vi "AFG3352X.constructor.vi"(0 "name":string, 2 "data in":string, 5 "error in (no error)":errorcluster) -> (14 "i ref out":refnum<vi>, 16 "data out":string, 19 "error out":errorcluster)   [LabVIEW 2014, in "AFG3352X.lvlib"]
doc: "Constructor of the AG33XXX class.\n\nLicense Agreement for this software:\n\nCopyright (C)\nGesellschaft für Schwerionenforschung, GSI\nPlanckstr. 1\n64291 Darmstadt\nGermany\n\nContact: D.Beck@gsi.de \n\nThis program is free software; you can redistribute it and/or modify it under the terms of the \nGNU General Public License as published by the Free Software Foundation; either version 2 of \nthe license, or (at your option) any later version.\n\nThis program is distributed in the hope that it will be useful, but WITHOUT ANY WARRANTY; \nwithout even the implied warranty of MERCHANTABILITY or FITNESS FOR A PARTICULAR PURPOSE. See the GNU General License for more details (http://www.gnu.org).\n\nGesellschaft für Schwerionenforschung, GSI\nPlanckstr. 1, 64291 Darmstadt, Germany\nFor all questions and ideas contact: M.Richter@gsi.de, H.Brand@gsi.de or D.Beck@gsi.de.\nLast update: 16-JUN-2004"
uses:
  AFG3352X.lvlib
  CS_Core/CSApplicationBaseClasses/DeviceBase/DeviceBase.myEventNames.ctl
  CS_Core/CSApplicationBaseClasses/AFGBase/AFGBase.myEventNames.ctl
  CS_Core/CSSystem/CSSystemLib/CSSystemLib.lvlib
  CS_Core/CSApplicationBaseClasses/AFGBase/AFGBase.lvlib
  CS_Core/CSApplicationBaseClasses/DeviceBase/DeviceBase.lvlib
  CS_Core/CSObj/CSObj.lvlib
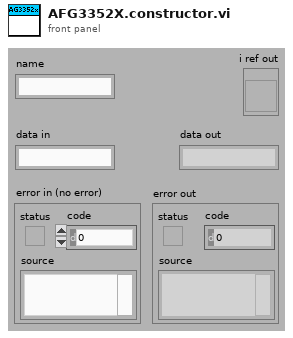
[diagram p1: front panel]
types:
  T1 = enum16{"SetAttribute", "GetAttribute", "CreateAttribute", "DestroyAttribute", "DestroyAllAtributes"}
  T2 = typedef "AFGBase.lvlib/AFGBase.myEventNames.ctl" = enum16{"lvmsg://SetFrequency", "lvmsg://GetFrequency", "lvmsg://SetAmplitude", "lvmsg://GetAmplitude", "lvmsg://SetPhase", "lvmsg://GetPhase", "lvmsg://SetDCOffset", "lvmsg://GetDCOffset", "lvmsg://SetWaveformType", "lvmsg://GetWaveformType", "lvmsg://SetOutputEnabled", "lvmsg://GetOutputEnabled", "lvmsg://SetWaveform", "lvmsg://GetWaveform", "lvmsg://SetTrigger", "lvmsg://GetTrigger", "lvmsg://SetWaveformParams", "lvmsg://GetWaveformParams"}
  T3 = typedef "DeviceBase.lvlib/DeviceBase.myEventNames.ctl" = enum16{"lvmsg://Initialize", "lvmsg://Close", "lvmsg://Configure", "lvmsg://Reset", "lvmsg://IDQuery"}
  T4 = typedef "CSObj.lvlib/CSObj.i attribute.ctl" = cluster{"VI Refnum":refnum<vi>, "Front Panel Ref":refnum<vi>, "semaphore":T5, "date of birth":dbl, "ageID":i32, "systemID":i32, "classID":i32, "conditionID":i32, "DefaultPanelType":u16}
  T5 = typedef "Semaphore RefNum" = refnum<k1>
  T6 = typedef "AFG3352X.lvlib/AFG3352X.i attribute.ctl" = cluster{"Act2ndValues":cluster{"frequency":dbl, "amplitude":dbl, "phase":dbl, "DCOffset":dbl, "waveformType":T7, "enableOutput":bool, "trigger":i16[], "serviceIDs":cluster{"frequencyID":i32, "amplitudeID":i32, "phaseID":i32, "DCOffsetID":i32, "waveformTypeID":i32, "enableOutputID":i32, "triggerID":i32}, "waveform":cluster{"data":waveform(dbl), "gain":dbl, "offset":dbl, "repetitionRate":dbl, "sampleRate":dbl}}, "Nom2ndValues":cluster{"frequency":dbl, "amplitude":dbl, "phase":dbl, "DCOffset":dbl, "waveformType":T7, "enableOutput":bool, "trigger":i16[], "serviceIDs":cluster{"frequencyID":i32, "amplitudeID":i32, "phaseID":i32, "DCOffsetID":i32, "waveformTypeID":i32, "enableOutputID":i32, "triggerID":i32}, "waveform":cluster{"data":waveform(dbl), "gain":dbl, "offset":dbl, "repetitionRate":dbl, "sampleRate":dbl}}, "DefaultChannel":i32, "ActAddValues":cluster{"Mode1":u16, "serviceIDs":cluster{"Mode1ID":i32, "Mode2ID":i32, "Burst1ID":i32, "Burst2ID":i32}, "Mode2":u16, "Burst1":i32, "Burst2":i32}, "NomAddValues":cluster{"Mode1":u16, "serviceIDs":cluster{"Mode1ID":i32, "Mode2ID":i32, "Burst1ID":i32, "Burst2ID":i32}, "Mode2 2":u16, "Burst1":i32, "Burst2":i32}, "enableBurstMode":bool}
  T7 = typedef "AFGBase.lvlib/AFGBase.waveformType.ctl" = enum16{"sine", "square", "ramp", "pulse", "noise", "DC", "arbitrary", "triangle", "ramp_up", "ramp_down", "amplitude modulation"}
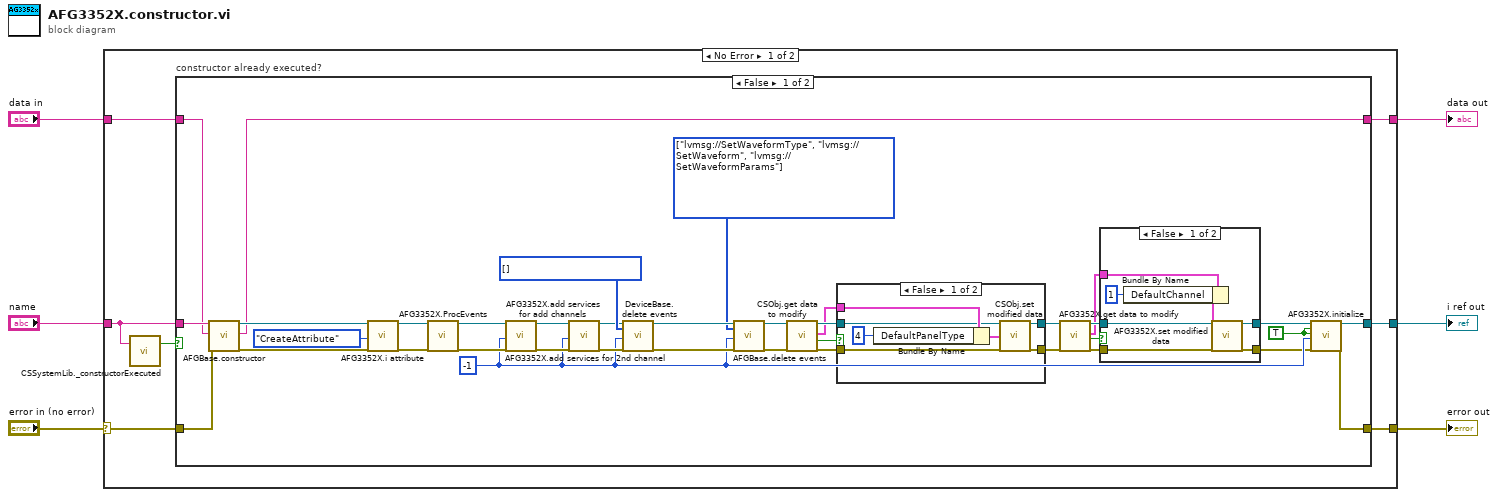
[diagram p0: block diagram]
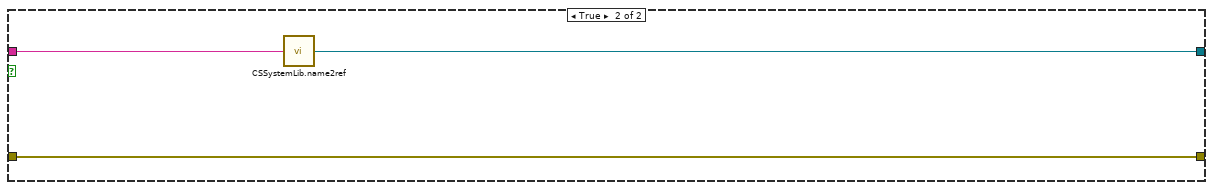
[diagram p4: hidden frame]
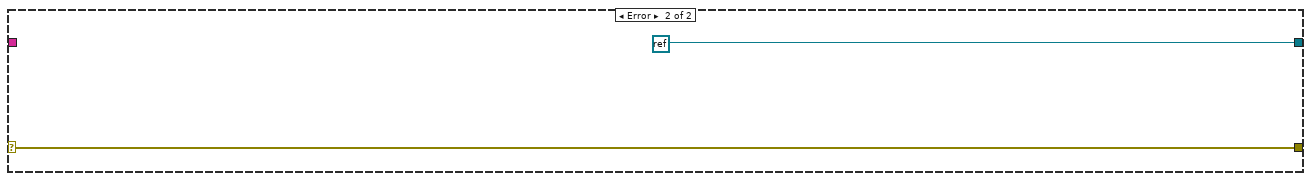
[diagram p5: hidden frame]
diagram:
  n1 = case shown="No Error" "error in (no error)" {
    selector: "error in (no error)" -> [w11 w72]
    tunnel: "name" -> [w10 _]
    tunnel: [w13 refnum<k0> refnum] -> w5
    tunnel: [w12 w72] -> w4
    tunnel: "data in" -> [w8 _]
    tunnel: [w7 _] -> w1
    frame No Error {
      n2 = call "CSSystemLib._constructorExecuted.vi"("name"=w10) -> ("constructor executed?"=w9:bool)  [unwired: 18 in]
      n3 = case "constructor already executed?" shown="False" w9 {
        tunnel: w10 -> [w47 w71]
        tunnel: [w38 w70] -> w13
        tunnel: [w37 w69] -> w12
        tunnel: w11 -> [w44 w69]
        tunnel: w8 -> [w43 _]
        tunnel: [w35 _] -> w7
        frame False {
          w39 = T2[] [enum."lvmsg://SetWaveformType", enum."lvmsg://SetWaveform", enum."lvmsg://SetWaveformParams"] items=["lvmsg://SetFrequency", "lvmsg://GetFrequency", "lvmsg://SetAmplitude", "lvmsg://GetAmplitude", "lvmsg://SetPhase", "lvmsg://GetPhase", "lvmsg://SetDCOffset", "lvmsg://GetDCOffset", "lvmsg://SetWaveformType", "lvmsg://GetWaveformType", "lvmsg://SetOutputEnabled", "lvmsg://GetOutputEnabled", "lvmsg://SetWaveform", "lvmsg://GetWaveform", "lvmsg://SetTrigger", "lvmsg://GetTrigger", "lvmsg://SetWaveformParams", "lvmsg://GetWaveformParams"] ("events")
          w42 = T3[] [] items=["lvmsg://Initialize", "lvmsg://Close", "lvmsg://Configure", "lvmsg://Reset", "lvmsg://IDQuery"] ("events")
          w36 = TRUE ("queryID")
          w22 = -1 ("ms timeout (10000)")
          n4 = call "AFGBase.constructor.vi"("name"=w47, "data in"=w43, "error in (no error)"=w44) -> ("i ref out"=w50:refnum<vi>, "data out"=w35:string, "error out"=w49:errorcluster)  [unwired: 14 in]
          n5 = call "AFG3352X.i attribute.vi"("VI Refnum"=w50, "Action"=T1."CreateAttribute", "error in (no error)"=w49) -> ("VI Refnum out"=w46:refnum<vi>, "error out"=w45:errorcluster)  [unwired: 14 in, 1 out]
          n6 = call "AFG3352X.ProcEvents.vi"("i ref in"=w46, "error in (no error)"=w45) -> ("i ref out"=w33:refnum<vi>, "error out"=w34:errorcluster)  [unwired: 16 in]
          n7 = call "AFG3352X.add services for 2nd channel.vi"("i ref in"=w33, "ms timeout (10000)"=w22, "error in (no error)"=w34) -> ("i ref out"=w26:refnum<vi>, "error out"=w23:errorcluster)  [unwired: 14 in, 1 out]
          n8 = call "AFG3352X.add services for add channels.vi"("i ref in"=w26, "ms timeout (10000)"=w22, "error in (no error)"=w23) -> ("i ref out"=w25:refnum<vi>, "error out"=w24:errorcluster)  [unwired: 14 in, 1 out]
          n9 = call "DeviceBase.delete events.vi"("i ref in"=w25, "events"=w42, "ms timeout (10000)"=w22, "error in (no error)"=w24) -> ("i ref out"=w41:refnum<vi>, "error out"=w40:errorcluster)  [unwired: 13 in, 1 out]
          n10 = call "AFGBase.delete events.vi"("i ref in"=w41, "events"=w39, "ms timeout (10000)"=w22, "error in (no error)"=w40) -> ("i ref out"=w28:refnum<vi>, "error out"=w27:errorcluster)  [unwired: 13 in, 1 out]
          n11 = call "CSObj.get data to modify.vi"("i ref in"=w28, "error in (no error)"=w27) -> ("i ref out"=w31:refnum<vi>, "i attribute"=w29:T4, "timed out"=w32:bool, "error out"=w30:errorcluster)  [unwired: 14 in]
          n12 = case shown="False" w32 {
            tunnel: [w64 w68] -> w20
            tunnel: w31 -> [w65 w68]
            tunnel: [w62 w67] -> w21
            tunnel: w30 -> [w63 w67]
            tunnel: w29 -> [w66 _]
            frame False {
              n13 = Bundle By Name(cluster=w66, "DefaultPanelType"=u16 4) -> (w61:T4)
              n14 = call "CSObj.set modified data.vi"("i ref in"=w65, "i attribute"=w61, "error in (no error)"=w63) -> ("i ref out"=w64:refnum<vi>, "error out"=w62:errorcluster)  [unwired: 15 in]
            }
            frame True {
            }
          }
          n15 = call "AFG3352X.get data to modify.vi"("i ref in"=w20, "error in (no error)"=w21) -> ("i ref out"=w17:refnum<vi>, "i attribute"=w14:T6, "timed out"=w15:bool, "error out"=w19:errorcluster)  [unwired: 14 in]
          n16 = case shown="False" w15 {
            tunnel: w19 -> [w57 w58]
            tunnel: [w56 w58] -> w18
            tunnel: w17 -> [w55 w59]
            tunnel: [w54 w59] -> w16
            tunnel: w14 -> [w53 _]
            frame False {
              n17 = Bundle By Name(cluster=w53, "DefaultChannel"=1) -> (w52:T6)
              n18 = call "AFG3352X.set modified data.vi"("i ref in"=w55, "i attribute"=w52, "error in (no error)"=w57) -> ("i ref out"=w54:refnum<vi>, "error out"=w56:errorcluster)  [unwired: 15 in]
            }
            frame True {
            }
          }
          n19 = call "AFG3352X.initialize.vi"("i ref in"=w16, "queryID"=w36, "resetDevice"=w36, "ms timeout (10000)"=w22, "error in (no error)"=w18) -> ("i ref out"=w38:refnum<vi>, "error out"=w37:errorcluster)  [unwired: 11 in, 2 out]
        }
        frame True {
          n20 = call "CSSystemLib.name2ref.vi"("name"=w71) -> ("obj refnum"=w70:refnum<vi>)
        }
      }
    }
    frame Error {
    }
  }
  "i ref out" <- w5
  "error out" <- w4
  "data out" <- w1
